vi "Get Reference to First Open Parent.vi"() -> (1 "Open Parent's Name":string, 2 "vi reference (close me!)":refnum<vi>)   [LabVIEW 2014]
doc: "This VI finds the first parent above this VI in the calling tree that has an open front panel and returns it's reference. If the reference is invalid that no parents are open.\nYou must close this reference!"
panel:
  # "This VI finds the first parent above this VI in the calling tree\nthat has an open front panel and returns it's reference.\nIf the reference is invalid that no parents are open.\nYou must close this reference!"
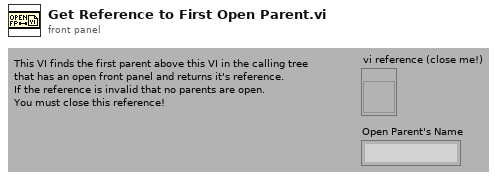
[diagram p1: front panel]
types:
  T1 = enum32{"Invalid", "Standard", "Closed", "Hidden", "Minimized", "Maximized"}
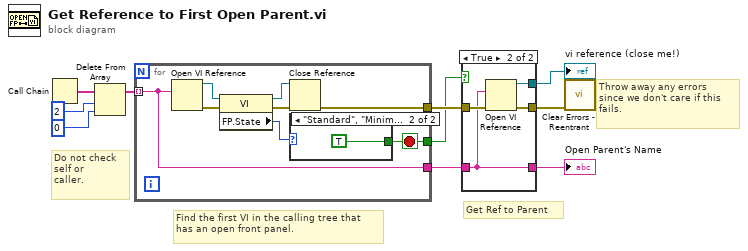
[diagram p0: block diagram]
diagram:
  # "Do not check\nself or\ncaller."
  # "Get Ref to Parent"
  # "Find the first VI in the calling tree that\nhas an open front panel."
  # "Throw away any errors\nsince we don't care if this\nfails."
  n1 = Call Chain() -> (call chain=w8:string[])
  n2 = Delete From Array(array=w8, length=2, index=0) -> (array with subset deleted=w9:string[])  [unwired: 1 out]
  n3 = for {
    tunnel: w9 -> [w16] mode=indexing
    tunnel: [w16] -> w2
    tunnel: [w11] -> w3
    tunnel: [w13] -> w5
    stop <- w11 stop-if-true
    n4 = Open VI Reference(vi path=w16) -> (vi reference=w18:refnum<vi>, error out=w15:errorcluster)  [unwired: 1 in, 4 out]
    n5 = property class="VI"(reference=w18, error in=w15) -> (reference out=w17:refnum<vi>, error out=w14:errorcluster, "FP.State"=w12:T1)
    n6 = Close Reference(reference=w17, error in (no error)=w14) -> (error out=w13:errorcluster)
    n7 = case shown="\"Standard\", \"Minimized\", \"Maximized\"" w12 {
      tunnel: [_ TRUE] -> w11
      frame Default {
        # "Not Open"
      }
      frame "Standard", "Minimized", "Maximized" {
      }
    }
  }
  n8 = case shown="True" w3 {
    tunnel: w2 -> [_ w21]
    tunnel: [_ w24] -> w4
    tunnel: w5 -> [w20 w23]
    tunnel: [w20 w22] -> w6
    tunnel: [_ w21] -> w7
    frame False {
    }
    frame True {
      n9 = Open VI Reference(vi path=w21, error in (no error)=w23) -> (vi reference=w24:refnum<vi>, error out=w22:errorcluster)  [unwired: 4 out]
    }
  }
  "vi reference (close me!)" <- w4
  "Open Parent's Name" <- w7
  n10 = call "Clear Errors - Reentrant.vi"("error in (no error)"=w6) -> ()  [unwired: 7 out]
